vi "kalman gain.vi"(9 "Pk|k-1":T1, 10 "S^-1":T1) -> (3 "K_k":T1)   [LabVIEW 2017]
uses:
  <vilib>/Analysis/Matrix/Datatypes/RealMatrix.ctl
  <vilib>/Analysis/Matrix/NI_Matrix.lvlib
  <vilib>/Analysis/Matrix/Numeric/Multiply/Multiply - RM,RM.vi
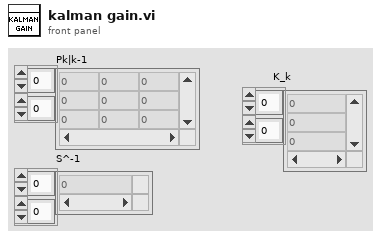
[diagram p1: front panel]
types:
  T1 = typedef "NI_Matrix.lvlib/RealMatrix.ctl" = dbl[][]
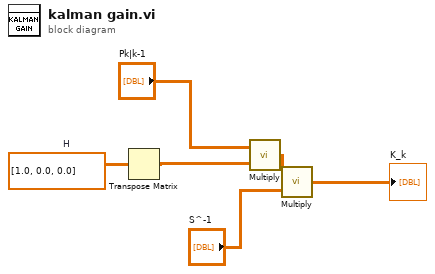
[diagram p0: block diagram]
diagram:
  w3 = T1 [[1.0, 0.0, 0.0]]  # H
  n1 = Transpose Matrix(1:w3) -> (0:w6:T1)
  n2 = call-poly <vilib>:"Multiply.vi"("Real Matrix B"=w6, "Real Matrix A"="Pk|k-1") -> ("A * B"=w5:T1)
  n3 = call-poly <vilib>:"Multiply.vi"("Real Matrix B"="S^-1", "Real Matrix A"=w5) -> ("A * B"=→"K_k":T1)
